vi "createEvents.vi"(8 "error in (no error)":errorcluster, 11 "ScriptEdEvents in":refnum<class "ScriptEdEvents.lvclass">) -> (0 "error out":errorcluster, 3 "ScriptEdEvents out":refnum<class "ScriptEdEvents.lvclass">)   [LabVIEW 2011, in "Views.lvlib" / "ScriptEditor.lvlib" / "ScriptEdEvents.lvclass"]
doc: "ScriptEdEvents Create.\n\nUsed to communicate between the Experiment Runner and Script Editor.\nopen/close/save scripts."
uses:
  ScriptEdEvents.lvclass
  ScriptEdEvents.lvclass/ScriptEdEvents.ctl
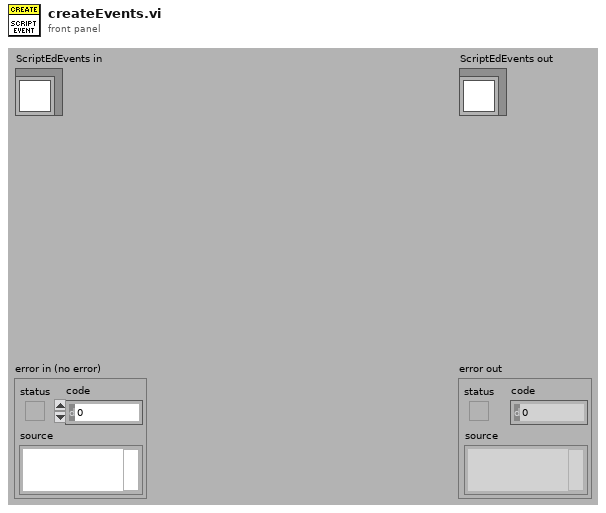
[diagram p1: front panel]
types:
  T1 = cluster{"eventId":enum16{"Open", "Save", "Close"}, "data":variant}
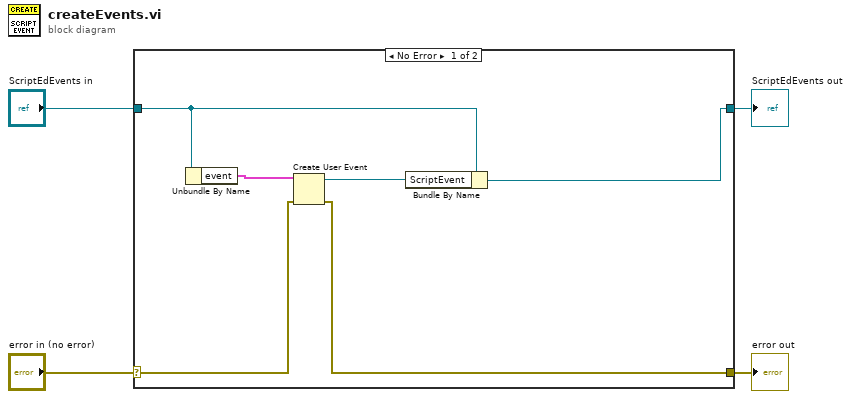
[diagram p0: block diagram]
diagram:
  n1 = case shown="No Error" "error in (no error)" {
    selector: "error in (no error)" -> [w6 w12]
    tunnel: [w5 w12] -> w3
    tunnel: [w8 w11] -> w1
    tunnel: "ScriptEdEvents in" -> [w9 w11]
    frame No Error {
      n2 = Unbundle By Name(w9) -> ("event"=w10:T1)
      n3 = Create User Event(user event datatype=w10, error in=w6) -> (user event=w7:refnum<user-event>, error out=w5:errorcluster)
      n4 = Bundle By Name(cluster=w9, "ScriptEvent"=w7) -> (w8:refnum<class "ScriptEdEvents.lvclass">)
    }
    frame Error {
    }
  }
  "error out" <- w3
  "ScriptEdEvents out" <- w1
